vi "TestMFCFill.vi"() -> ()   [LabVIEW 2018]
panel:
  out "Pressure Error":errorcluster
  in  "Fill Time (s)":dbl=10.0
  out "3He Pressure (Torr)":dbl
  out "MFC Error":errorcluster
  in  "Tare":bool
  in  "Stop":bool
  in  "Fill":bool
  in  "SetPoint (Torr)":dbl
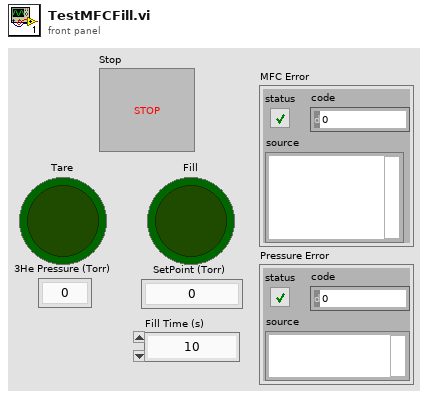
[diagram p1: front panel]
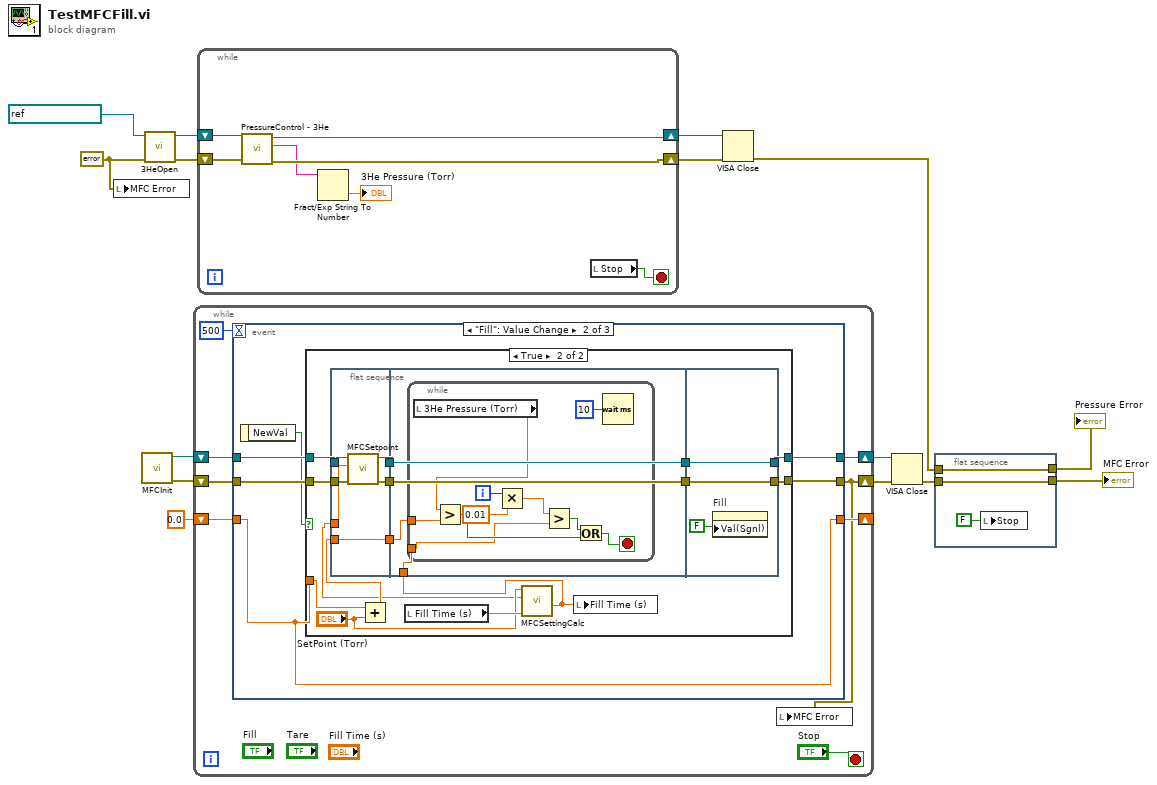
[diagram p0: block diagram]
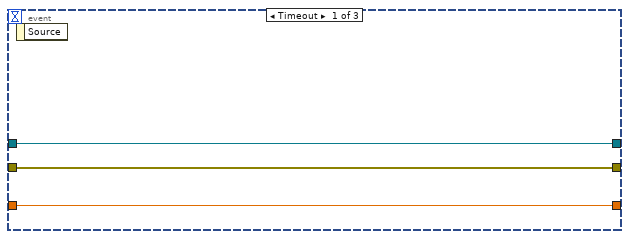
[diagram p2: hidden frame]
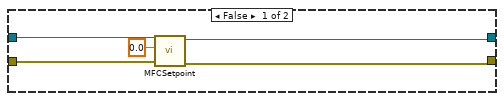
[diagram p3: hidden frame]
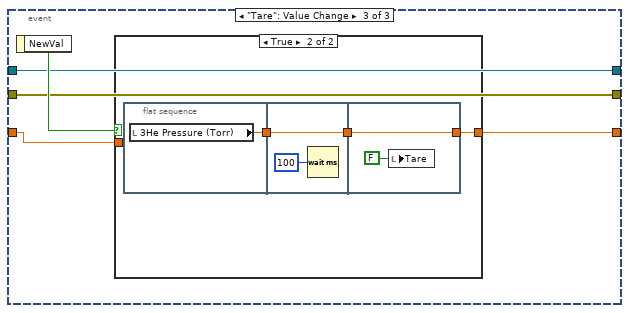
[diagram p4: hidden frame]
diagram:
  w1 = errorcluster {"status"=FALSE, "code"=0, "source"=""} ("error in (no error) 2")
  n1 = local write "MFC Error"(w1) -> ()
  n2 = call "MFCInit.vi"() -> ("MFC error out"=w12:errorcluster, "MFC VISA out"=w13:refnum<visa-resource-name>)  [unwired: 10 in]
  n3 = call "3HeOpen.vi"("error in (no error)"=w1, "VISA resource name"=refnum<visa-resource-name> "3HePressure" ("Pressure Gauge")) -> ("error out"=w9:errorcluster, "VISA resource name out"=w10:refnum<visa-resource-name>)  [unwired: 8 in]
  n4 = while {
    shift-right: [w20] -> w14
    shift-left: w13 -> [w22]
    shift-right: [w16] -> w15
    shift-left: w12 -> [w23]
    shift-right: [w18] -> _
    shift-left: 0.0 ("3He Pressure") -> [w17]
    stop <- "Stop" stop-if-true
    n5 = event shown="[1] \"Fill\": Value Change" {
      selector: _ -> [_ _ _]
      dyn-events: _ -> [_ _ _]
      timeout: 500 -> [_ _ _]
      tunnel: w23 -> [w26 w32 w78]
      tunnel: [w26 w29 w78] -> w16
      tunnel: w22 -> [w25 w31 w79]
      tunnel: [w25 w30 w79] -> w20
      tunnel: [w24 w27 w77] -> w18
      tunnel: w17 -> [w24 w27 w76]
      event Timeout {
        n6 = event-data() -> ()  [unwired: 1 in, 1 out]
      }
      event "Fill": Value Change {
        n7 = event-data() -> ("NewVal"=w28:bool)  [unwired: 1 in]
        n8 = case shown="True" w28 {
          tunnel: w32 -> [w37 w52]
          tunnel: w31 -> [w36 w51]
          tunnel: [w35 w50] -> w30
          tunnel: [w34 w49] -> w29
          tunnel: w27 -> [_ w43]
          frame False {
            n9 = call "MFCSetpoint.vi"("MFC error in"=w37, "MFC setpoint"=0.0, "MFC VISA in"=w36) -> ("MFC error out"=w34:errorcluster, "MFC VISA out"=w35:refnum<visa-resource-name>)  [unwired: 7 in]
          }
          frame True {
            n10 = flat-sequence {
              tunnel: w52 -> [w58]
              tunnel: w51 -> [w57]
              tunnel: [w56] -> w48
              tunnel: [w55] -> w47
              tunnel: w39 -> [w54]
              tunnel: w42 -> [w53]
              tunnel: [w53] -> w44
              tunnel: w48 -> [w62]
              tunnel: w47 -> [w61]
              tunnel: [w62] -> w46
              tunnel: [w61] -> w45
              tunnel: w44 -> [w60]
              tunnel: w38 -> [w59]
              tunnel: [w74] -> w49
              tunnel: [w75] -> w50
              tunnel: w46 -> [w75]
              tunnel: w45 -> [w74]
              frame #0 {
                n11 = call "MFCSetpoint.vi"("MFC error in"=w58, "MFC setpoint"=w54, "MFC VISA in"=w57) -> ("MFC error out"=w55:errorcluster, "MFC VISA out"=w56:refnum<visa-resource-name>)  [unwired: 7 in]
              }
              frame #1 {
                n12 = while {
                  tunnel: w60 -> [w72]
                  tunnel: w59 -> [w63]
                  i -> [w66]
                  stop <- w70 stop-if-true
                  n13 = local read "3He Pressure (Torr)"() -> (w71:dbl)
                  n14 = Greater?(x=w71, y=w72) -> (0:w69:bool)
                  n15 = Multiply(x=w66, y=0.01) -> (x*y=w65:dbl)
                  n16 = Greater?(x=w65, y=w63) -> (0:w67:bool)
                  n17 = Or(x=w67, y=w69) -> (x .or. y?=w70:bool)
                  n18 = Wait (ms)(milliseconds to wait=u32 10) -> ()  [unwired: 1 out]
                }
              }
              frame #2 {
                n19 = property on="Fill" class="Bool (strict)"("Val(Sgnl)"=FALSE ("Value (Signaling)")) -> ()  [unwired: 2 in, 2 out]
              }
            }
            n20 = Add(x=w43, y="SetPoint (Torr)") -> (x+y=w42:dbl)
            n21 = local read "Fill Time (s)"() -> (w41:dbl)
            n22 = call "MFCSettingCalc.vi"("Fill Time (s)"=w41, "SetPoint"="SetPoint (Torr)") -> ("Time (s)"=w38:dbl, "MFC Setting"=w39:dbl)  [unwired: 8 in]
            n23 = local write "Fill Time (s)"(w38) -> ()
          }
        }
      }
      event "Tare": Value Change {
        n24 = event-data() -> ("NewVal"=w80:bool)  [unwired: 1 in]
        n25 = case shown="True" w80 {
          tunnel: [w81 w84] -> w77
          tunnel: w76 -> [w81 _]
          frame False {
          }
          frame True {
            n26 = flat-sequence {
              tunnel: [w85] -> w83
              tunnel: w83 -> [w87]
              tunnel: [w87] -> w82
              tunnel: [w89] -> w84
              tunnel: w82 -> [w89]
              frame #0 {
                n27 = local read "3He Pressure (Torr)"() -> (w85:dbl)
              }
              frame #1 {
                n28 = Wait (ms)(milliseconds to wait=u32 100) -> ()  [unwired: 1 out]
              }
              frame #2 {
                n29 = local write "Tare"(FALSE ("Tare")) -> ()
              }
            }
          }
        }
      }
    }
    n30 = local write "MFC Error"(w16) -> ()
  }
  n31 = while {
    shift-right: [w92] -> w5
    shift-left: w9 -> [w95]
    shift-right: [w93] -> w4
    shift-left: w10 -> [w94]
    stop <- w96 stop-if-true
    n32 = call "PressureControl - 3He.vi"("error in (no error)"=w95, "VISA resource name"=w94) -> ("error out"=w92:errorcluster, "3HePressure (Torr)"=w91:string, "VISA resource name out"=w93:refnum<visa-resource-name>)  [unwired: 7 in]
    n33 = Fract/Exp String To Number(string=w91) -> (number=→"3He Pressure (Torr)":dbl)  [unwired: 3 in, 1 out]
    n34 = local read "Stop"() -> (w96:bool)
  }
  n35 = VISA Close(VISA resource name=w4, error in (no error)=w5) -> (error out=w3:errorcluster)
  n36 = VISA Close(VISA resource name=w14, error in (no error)=w15) -> (error out=w8:errorcluster)
  n37 = flat-sequence {
    tunnel: w8 -> [w99]
    tunnel: [w99] -> w7
    tunnel: w3 -> [w97]
    tunnel: [w97] -> w2
    frame #0 {
      n38 = local write "Stop"(FALSE ("Stop")) -> ()
    }
  }
  "MFC Error" <- w7
  "Pressure Error" <- w2
